vi "SQL_聚集索引.vi"(6 "字段名":string="DELETE FROM table_name", 7 "功能":enum16{"CREATE", "DELETE"}(ring), 8 "error in (no error)":errorcluster, 9 "索引名":string="DELETE FROM table_name", 10 "表名":string="DELETE FROM table_name", 11 "connection reference":T1) -> (0 "error out":errorcluster)   [LabVIEW 2014]
uses:
  <vilib>/addons/database/Connection.llb/Conn ObjectReference.ctl
  <vilib>/addons/database/Connection.llb/Conn Execute.vi
  <vilib>/addons/database/Recordset.llb/Rec Destroy - Connection.vi
  <vilib>/addons/database/NI_Database_API.lvlib
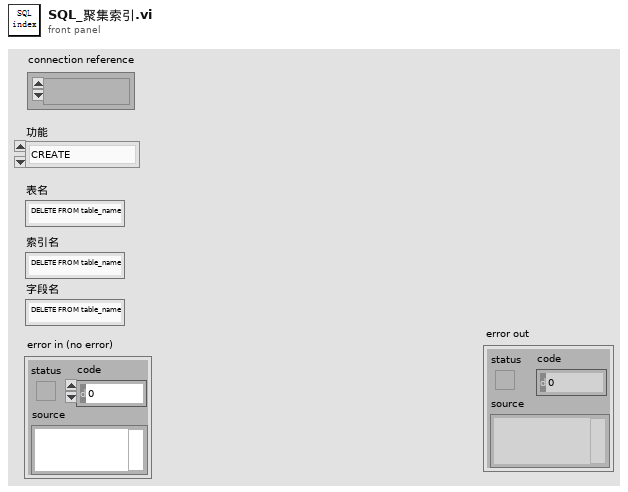
[diagram p1: front panel]
types:
  T1 = typedef "NI_Database_API.lvlib/Conn ObjectReference.ctl" = refnum<k1>
  T2 = typedef "NI_Database_API.lvlib/Rec ObjectReference.ctl" = refnum<k1>
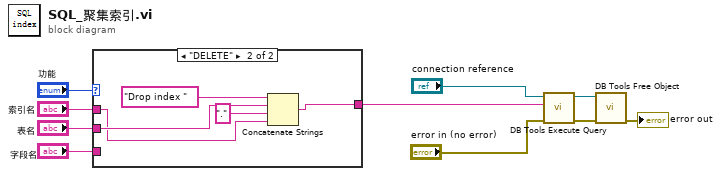
[diagram p0: block diagram]
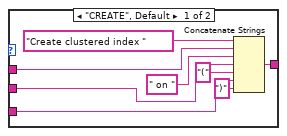
[diagram p2: hidden frame]
diagram:
  n1 = case shown="\"DELETE\"" "功能" {
    tunnel: "索引名" -> [w17 w20]
    tunnel: "表名" -> [w15 w22]
    tunnel: "字段名" -> [w13 _]
    tunnel: [w11 w19] -> w1
    frame "CREATE", Default {
      n2 = Concatenate Strings("Create clustered index " ("字符串"), w17, " on " ("字符串"), w15, "(" ("字符串"), w13, ")" ("字符串")) -> (w11:string)
    }
    frame "DELETE" {
      n3 = Concatenate Strings("Drop index " ("字符串"), w22, "." ("字符串"), w20) -> (w19:string)
    }
  }
  n4 = call-poly <vilib>:"DB Tools Execute Query.vi"("error in (no error)"="error in (no error)", "SQL query"=w1, "connection reference"="connection reference") -> ("error out"=w6:errorcluster, "recordset reference"=w7:T2)  [unwired: 5 in]
  n5 = call-poly <vilib>:"DB Tools Free Object.vi"("error in (no error)"=w6, "recordset reference"=w7) -> ("error out"=→"error out":errorcluster)  [unwired: 8 in, 1 out]
